vi "CheckDiskSpace.vi"(8 "error in":errorcluster, 11 "path":path) -> (0 "error out":errorcluster, 1 "Tweet text":string)   [LabVIEW 2014]
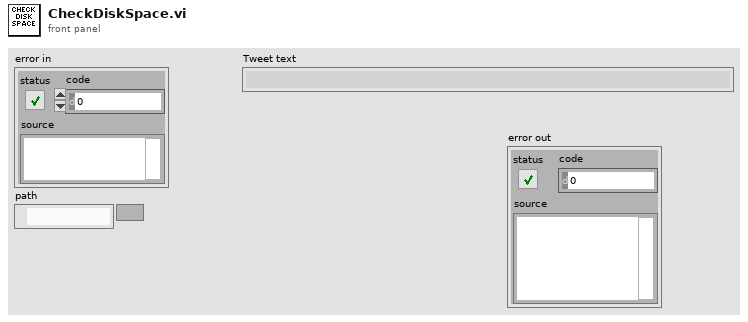
[diagram p1: front panel]
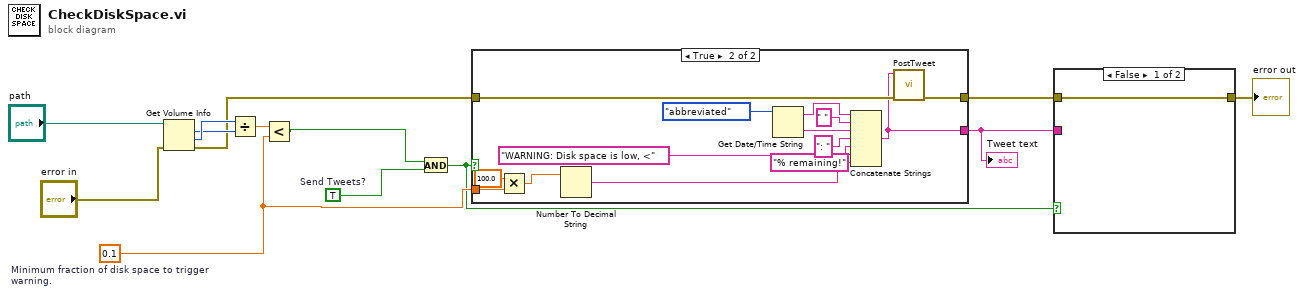
[diagram p0: block diagram]
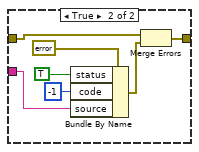
[diagram p2: hidden frame]
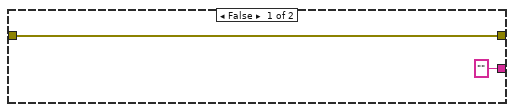
[diagram p3: hidden frame]
diagram:
  w2 = 0.1  # Minimum fraction of disk space to trigger warning.
  w5 = TRUE  # Send Tweets?
  n1 = Get Volume Info(8:"error in", 11:"path") -> (0:w3:errorcluster, 1:w8:i64, 2:w7:i64)  [unwired: 3 out]
  n2 = Divide(x=w8, y=w7) -> (x/y=w6:dbl)
  n3 = Less?(x=w6, y=w2) -> (x < y?=w4:bool)
  n4 = And(x=w4, y=w5) -> (x .and. y?=w1:bool)
  n5 = case shown="True" w1 {
    tunnel: w3 -> [w15 w29]
    tunnel: [w15 w28] -> w11
    tunnel: ["" w26] -> w13
    tunnel: w2 -> [_ w20]
    frame False {
    }
    frame True {
      n6 = Multiply(x=100.0, y=w20) -> (x*y=w18:dbl)
      n7 = Number To Decimal String(number=w18) -> (decimal integer string=w17:string)  [unwired: 1 in]
      n8 = Get Date/Time String(date format (0)=enum16{"short", "long", "abbreviated"}."abbreviated") -> (date string=w27:string, time string=w24:string)  [unwired: 2 in]
      n9 = Concatenate Strings(w27, " " ("string"), w24, ": " ("string"), "WARNING: Disk space is low, <" ("Tweet"), w17, "% remaining!" ("string")) -> (w26:string)
      n10 = call "PostTweet.vi"("error in"=w29, "Tweet"=w26) -> ("error out"=w28:errorcluster)  [unwired: 9 in]
    }
  }
  "Tweet text" <- w13
  n11 = case shown="False" w1 {
    tunnel: w13 -> [_ w35]
    tunnel: [w30 w33] -> w12
    tunnel: w11 -> [w30 w34]
    frame False {
    }
    frame True {
      n12 = Bundle By Name(cluster=errorcluster {"status"=FALSE, "code"=0, "source"=""} ("error constant"), "status"=TRUE, "code"=-1, "source"=w35) -> (w32:errorcluster)
      n13 = Merge Errors(w34, w32) -> (w33:errorcluster)
    }
  }
  "error out" <- w12
